vi "Disconnect From Meter.vi"(0 "Location of FieldMax2Lib.dll in":path=path "C:/Windows/SysWOW64/FieldMax2Lib.dll", 1 "Meter ID in":i32) -> (7 "Location of FieldMax2Lib.dll out":path, 8 "Meter ID out":i32)   [LabVIEW 2018]
panel:
  # "This VI should be run at the end of the routine to close communications with the meter."
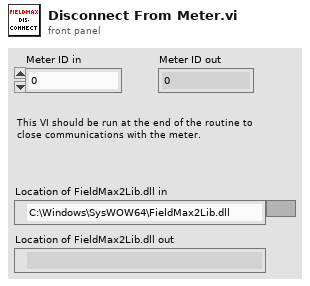
[diagram p1: front panel]
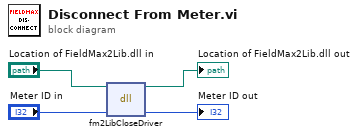
[diagram p0: block diagram]
diagram:
  n1 = dll-call lib="C:/Windows/System32/FieldMax2Lib.dll" fn="fm2LibCloseDriver" label="Close Driver"(path in="Location of FieldMax2Lib.dll in", "h"="Meter ID in") -> (path out=→"Location of FieldMax2Lib.dll out":path, "h"=→"Meter ID out":i32)  [unwired: 3 in, 1 out]
